vi "Configure Output Power.vi"(8 "error in (no error)":errorcluster, 10 "Output Power [dBm]":dbl, 11 "SigGen-SMBV in":refnum<class "SigGen-SMBV.lvclass">) -> (0 "error out":errorcluster, 3 "SigGen-SMBVout":refnum<class "SigGen-SMBV.lvclass">)   [LabVIEW 2020, in "SigGen-SMBV.lvclass"]
uses:
  SigGen-SMBV.lvclass
  C:/Sandbox/RF Bench/Source Code/WiSpry Test Framework/Instruments/Signal Generator/Signal Generator.lvclass
  C:/Sandbox/RF Bench/Source Code/WiSpry Test Framework/Instruments/Instrument.lvclass
  Signal Generator.lvclass/Signal Generator.ctl
  Instrument.lvclass/Instrument.ctl
  Signal Generator.lvclass
  Instrument.lvclass
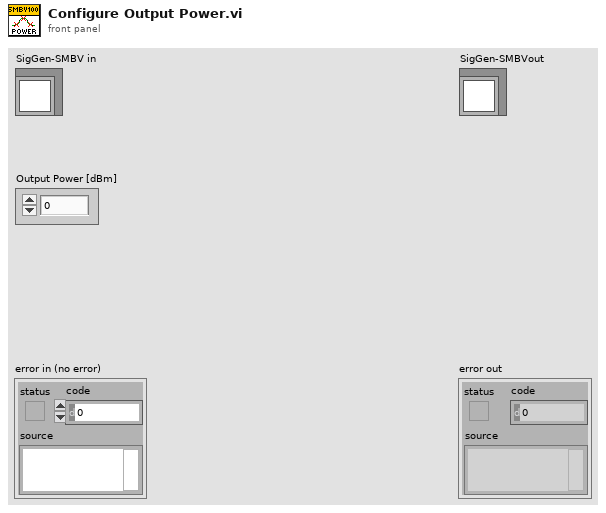
[diagram p1: front panel]
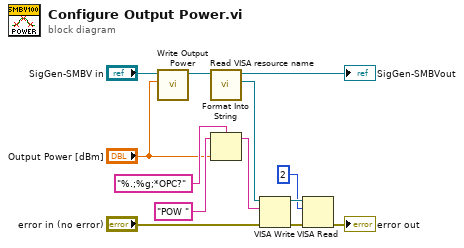
[diagram p0: block diagram]
diagram:
  n1 = call "Write Output Power.vi"("Output Power"="Output Power [dBm]", "Signal Generator in"="SigGen-SMBV in") -> ("Signal Generator out"=w8:refnum<class "SigGen-SMBV.lvclass">)  [unwired: 9 in]
  n2 = call "Read VISA resource name.vi"("Instrument in"=w8) -> ("VISA resource name"=w6:refnum<visa-resource-name>, "Instrument out"=→"SigGen-SMBVout":refnum<class "SigGen-SMBV.lvclass">)  [unwired: 9 in]
  n3 = Format Into String(format string="%.;%g;*OPC?", initial string="POW ", "Output Power [dBm]") -> (resulting string=w10:string)  [unwired: 1 in, 1 out]
  n4 = VISA Write(VISA resource name=w6, write buffer=w10, error in (no error)="error in (no error)") -> (VISA resource name out=w3:refnum<visa-resource-name>, error out=w4:errorcluster)  [unwired: 1 out]
  n5 = VISA Read(VISA resource name=w3, byte count=u32 2, error in (no error)=w4) -> (error out=→"error out":errorcluster)  [unwired: 3 out]
